vi "New Build Init Commands.vi"() -> (0 "SICK Commands":string[][](array[string]))   [LabVIEW 2009]
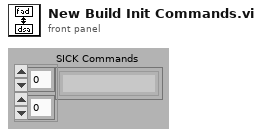
[diagram p1: front panel]
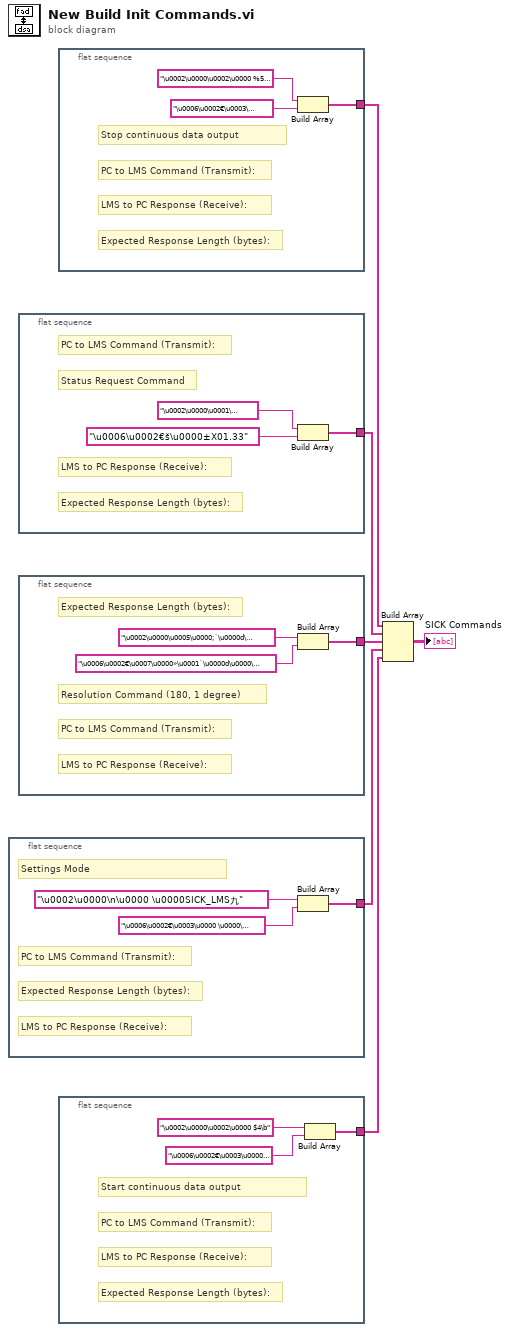
[diagram p0: block diagram]
diagram:
  n1 = flat-sequence {
    tunnel: [w7] -> w5
    frame #0 {
      # "Expected Response Length (bytes):"
      # "LMS to PC Response (Receive):"
      # "PC to LMS Command (Transmit):"
      # "Settings Mode"
      n2 = Build Array("\u0002\u0000\n\u0000 \u0000SICK_LMS九", "\u0006\u0002€\u0003\u0000 \u0000\u0010\u0016\n") -> (w7:string[])
    }
  }
  n3 = flat-sequence {
    tunnel: [w10] -> w2
    frame #0 {
      # "Expected Response Length (bytes):"
      # "LMS to PC Response (Receive):"
      # "PC to LMS Command (Transmit):"
      # "Status Request Command"
      n4 = Build Array("\u0002\u0000\u0001\u00001\u0015\u0012", "\u0006\u0002€š\u0000±X01.33") -> (w10:string[])
    }
  }
  n5 = flat-sequence {
    tunnel: [w13] -> w6
    frame #0 {
      # "Expected Response Length (bytes):"
      # "LMS to PC Response (Receive):"
      # "PC to LMS Command (Transmit):"
      # "Resolution Command (180, 1 degree)"
      n6 = Build Array("\u0002\u0000\u0005\u0000;´\u0000d\u0000—I", "\u0006\u0002€\u0007\u0000»\u0001´\u0000d\u0000\u0010[0") -> (w13:string[])
    }
  }
  n7 = flat-sequence {
    tunnel: [w16] -> w1
    frame #0 {
      # "Expected Response Length (bytes):"
      # "LMS to PC Response (Receive):"
      # "PC to LMS Command (Transmit):"
      # "Stop continuous data output"
      n8 = Build Array("\u0002\u0000\u0002\u0000 %5\b", "\u0006\u0002€\u0003\u0000 \u0000") -> (w16:string[])
    }
  }
  n9 = flat-sequence {
    tunnel: [w19] -> w4
    frame #0 {
      # "Expected Response Length (bytes):"
      # "LMS to PC Response (Receive):"
      # "PC to LMS Command (Transmit):"
      # "Start continuous data output"
      n10 = Build Array("\u0002\u0000\u0002\u0000 $4\b", "\u0006\u0002€\u0003\u0000 \u0000") -> (w19:string[])
    }
  }
  n11 = Build Array(w1, w2, w6, w5, w4) -> (→"SICK Commands":string[][])
